vi "Teste de timeout do servidor.vi"() -> ()   [LabVIEW 2016]
uses:
  <vilib>/addons/_JKI Toolkits/Caraya/classes/Assert/Assert.lvclass
  <vilib>/addons/_JKI Toolkits/Caraya/classes/Test/Test.lvclass
panel:
  out "error out":errorcluster
  in  "error in (no error)":errorcluster
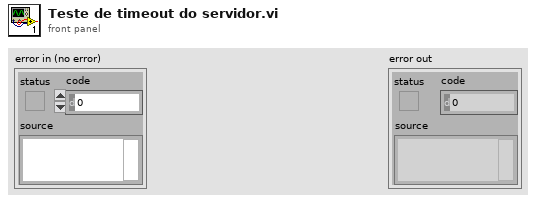
[diagram p1: front panel]
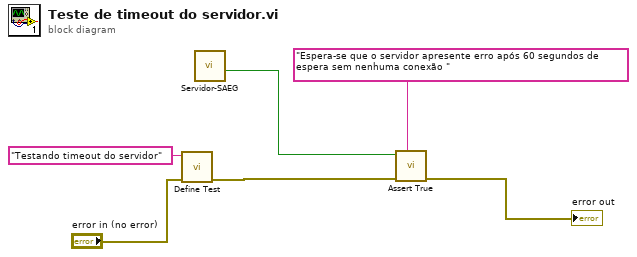
[diagram p0: block diagram]
diagram:
  n1 = call <vilib>:"Define Test.vi"("error in (no error)"="error in (no error)", "Label (VI Title)"="Testando timeout do servidor") -> ("error out"=w3:errorcluster)  [unwired: 9 in]
  n2 = call "Servidor-SAEG.vi"() -> ("status"=w6:bool)  [unwired: 10 in, 1 out]
  n3 = call <vilib>:"Assert True.vi"("Label"="Espera-se que o servidor apresente erro após 60 segundos de espera sem nenhuma conexão ", "error in (no error)"=w3, "True?"=w6) -> ("error out"=→"error out":errorcluster)  [unwired: 8 in]
